vi "sensor cmd memory crc16.vi"(7 "current_value":u16, 9 "length":u16, 10 "address":u32, 11 "device_handle":u32) -> (2 "function return":i32, 3 "device_handle out":u32, 5 "current_value out":u16)   [LabVIEW 2019, in "apdm.lvlib"]
doc: "APDM_EXPORT int apdm_sensor_cmd_memory_crc16(apdm_device_handle_t device_handle, const uint32_t address, const uint16_t length, uint16_t *current_value);"
uses:
  apdm.lvlib
  Lee Lab/CP FES Walking 2018/Code/Working/LabVIEW/apdm.dll
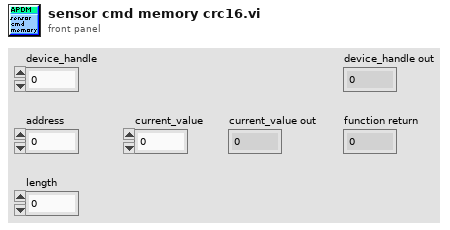
[diagram p1: front panel]
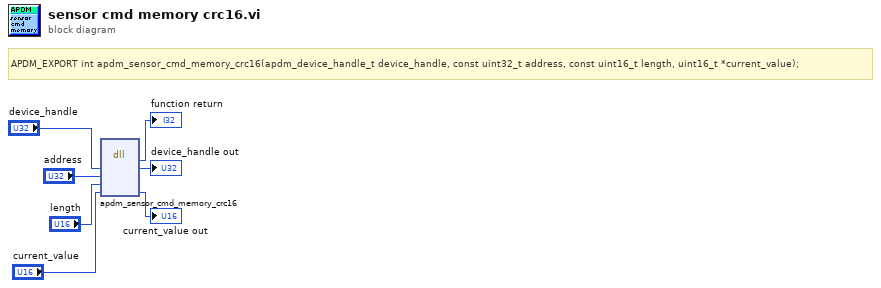
[diagram p0: block diagram]
diagram:
  # "APDM_EXPORT int apdm_sensor_cmd_memory_crc16(apdm_device_handle_t device_handle, const uint32_t address, const uint16_t length, uint16_t *current_value);"
  n1 = dll-call lib="C:/Users/jfalesi/Dropbox/Lee Lab/CP FES Walking 2018/Code/Working/LabVIEW/apdm.*" fn="apdm_sensor_cmd_memory_crc16"("device_handle"="device_handle", "address"="address", "length"="length", "current_value"="current_value") -> (→"function return":i32, "device_handle"=→"device_handle out":u32, "current_value"=→"current_value out":u16)  [unwired: 5 in, 2 out]
